vi "APS7050 Test.vi"() -> ()   [LabVIEW 2019, in "Wrappers.lvlib"]
uses:
  Wrappers.lvlib
  Controls/PS States.ctl
panel:
  out "Connect?":bool
  out "output cluster":T1
  in  "Setting":T2
  in  "stop":bool
  out "error out":errorcluster
  out "Measurement":dbl=nan
  in  "Enable Output":bool
  in  "Alias":string="ACPS"
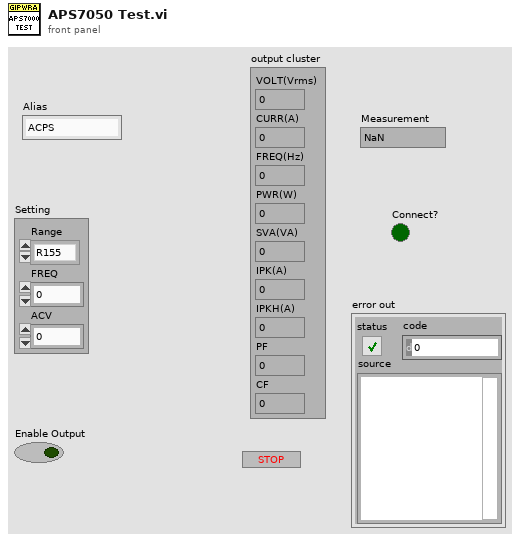
[diagram p1: front panel]
types:
  T1 = cluster{"VOLT(Vrms)":dbl, "CURR(A)":dbl, "FREQ(Hz)":dbl, "PWR(W)":dbl, "SVA(VA)":dbl, "IPK(A)":dbl, "IPKH(A)":dbl, "PF":dbl, "CF":dbl}
  T2 = cluster{"Range":enum16{"R155", "R310", "R600", "AUTO"}, "FREQ":dbl, "ACV":dbl}
  T3 = typedef "PS States.ctl" = enum16{"Init", "Config", "Enable Output", "Measure", "Close"}
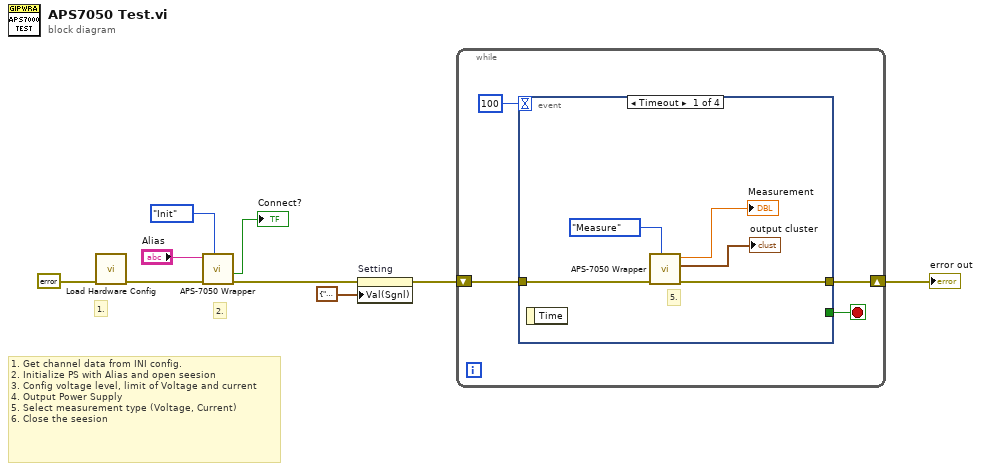
[diagram p0: block diagram]
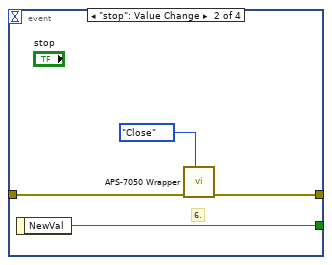
[diagram p2: hidden frame]
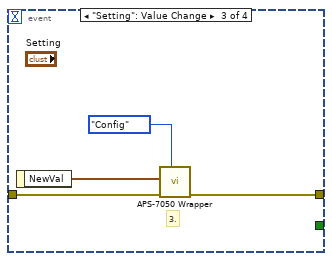
[diagram p3: hidden frame]
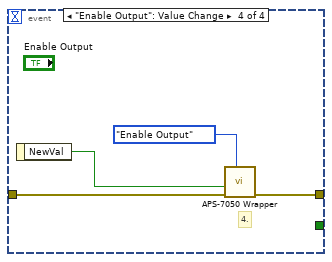
[diagram p4: hidden frame]
diagram:
  # "1. Get channel data from INI config.\n2. Initialize PS with Alias and open seesion \n3. Config voltage level, limit of Voltage and current\n4. Output Power Supply\n5. Select measurement type (Voltage, Current)\n6. Close the seesion"
  # "2."
  # "1."
  n1 = call "Load Hardware Config.vi"("error in"=errorcluster {"status"=FALSE, "code"=0, "source"=""}) -> ("error out"=w8:errorcluster)  [unwired: 10 in]
  n2 = call "APS-7050 Wrapper.vi"("States"=PS_States."Init", "error in"=w8, "Alias"="Alias") -> ("error out"=w3:errorcluster, "Connect?"=→"Connect?":bool)  [unwired: 5 in, 2 out]
  n3 = property on="Setting" class="Clust (strict)"(error in=w3, "Val(Sgnl)"=T2 {"Range"=enum."R155", "FREQ"=50.0, "ACV"=50.0} ("Setting")) -> (error out=w2:errorcluster)  [unwired: 1 in, 1 out]
  n4 = while {
    shift-right: [w11] -> w4
    shift-left: w2 -> [w12]
    stop <- w13 stop-if-true
    n5 = event shown="[0] Timeout" {
      selector: _ -> [_ _ _ _]
      dyn-events: _ -> [_ _ _ _]
      timeout: 100 -> [_ _ _ _]
      tunnel: [_ w22 _ _] -> w13
      tunnel: [w14 w19 w24 w28] -> w11
      tunnel: w12 -> [w15 w20 w25 w29]
      event Timeout {
        # "5."
        n6 = event-data() -> ()  [unwired: 1 in, 1 out]
        n7 = call "APS-7050 Wrapper.vi"("States"=PS_States."Measure", "error in"=w15) -> ("error out"=w14:errorcluster, "output cluster"=→"output cluster":T1, "Measurement"=→"Measurement":dbl)  [unwired: 6 in, 1 out]
      }
      event "stop": Value Change {
        # "6."
        n8 = event-data() -> ("NewVal"=w22:bool)  [unwired: 1 in]
        n9 = call "APS-7050 Wrapper.vi"("States"=PS_States."Close", "error in"=w20) -> ("error out"=w19:errorcluster)  [unwired: 6 in, 3 out]
      }
      event "Setting": Value Change {
        # "3."
        n10 = event-data() -> ("NewVal"=w23:T2)  [unwired: 1 in]
        n11 = call "APS-7050 Wrapper.vi"("States"=PS_States."Config", "error in"=w25, "Setting"=w23) -> ("error out"=w24:errorcluster)  [unwired: 5 in, 3 out]
      }
      event "Enable Output": Value Change {
        # "4."
        n12 = event-data() -> ("NewVal"=w27:bool)  [unwired: 1 in]
        n13 = call "APS-7050 Wrapper.vi"("States"=PS_States."Enable Output", "error in"=w29, "Enable Output"=w27) -> ("error out"=w28:errorcluster)  [unwired: 5 in, 3 out]
      }
    }
  }
  "error out" <- w4
